vi "Write Class to Error.vi"(8 "Error in":errorcluster, 11 "Calling Class":string) -> (0 "Error out":errorcluster)   [LabVIEW 2019, in "Logger.Error.lvlib" / "Logger.Error.lvclass"]
doc: "This VI includes a \"classification\" that helps to identify an error. Classification is typically done by a Specific Error Handler, but can be done manually using this VI. Classifications are typically consumed by a Central Error Handler. Classifications are represented by appending information to the error's source string."
uses:
  Logger.Error.lvclass
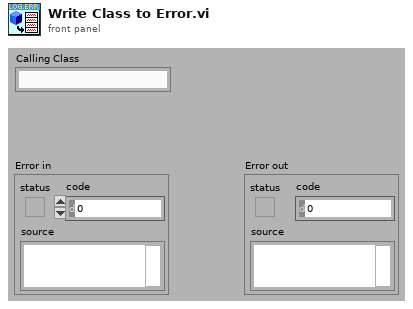
[diagram p1: front panel]
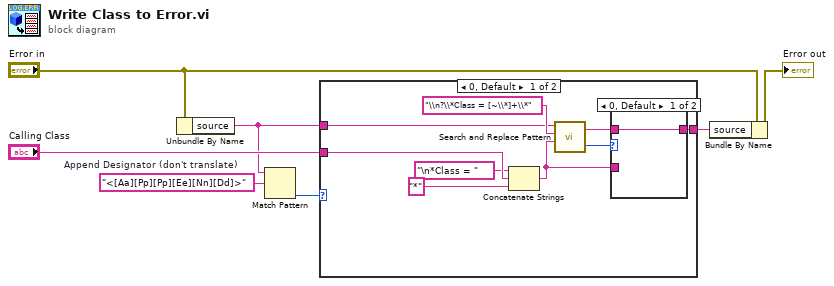
[diagram p0: block diagram]
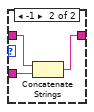
[diagram p2: hidden frame]
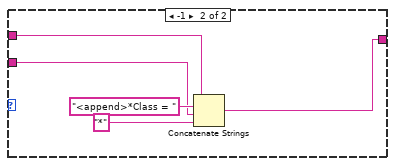
[diagram p3: hidden frame]
diagram:
  w5 = "<[Aa][Pp][Pp][Ee][Nn][Dd]>"  # Append Designator (don't translate)
  n1 = Unbundle By Name("Error in") -> ("source"=w3:string)
  n2 = Match Pattern(string=w3, regular expression=w5) -> (offset past match=w4:i32)  [unwired: 4 out]
  n3 = case shown="0, Default" w4 {
    tunnel: [w16 w21] -> w7
    tunnel: "Calling Class" -> [w12 w23]
    tunnel: w3 -> [w8 w22]
    frame 0, Default {
      n4 = Concatenate Strings("\n*Class = " ("string"), w12, "*" ("string")) -> (w9:string)
      n5 = call <vilib>:"Search and Replace Pattern.vi"("string"=w8, "regular expression (\"\")"="\\n?\\*Class = [~\\*]+\\*" ("regular expression (\"\")"), "replace string (\"\")"=w9) -> ("result string"=w15:string, "offset past match"=w14:i32)  [unwired: 2 out]
      n6 = case shown="0, Default" w14 {
        tunnel: w15 -> [w17 w18]
        tunnel: [w17 w20] -> w16
        tunnel: w9 -> [_ w19]
        frame 0, Default {
        }
        frame -1 {
          n7 = Concatenate Strings(w18, w19) -> (w20:string)
        }
      }
    }
    frame -1 {
      n8 = Concatenate Strings(w22, "<append>*Class = " ("string"), w23, "*" ("string")) -> (w21:string)
    }
  }
  n9 = Bundle By Name(cluster="Error in", "source"=w7) -> (→"Error out":errorcluster)
